vi "Get SMO Public API.vi"(8 "error in (no error)":errorcluster, 11 "Instrument.Amplifier in":refnum<class "Instrument.Amplifier.lvclass">) -> (0 "error out":errorcluster, 2 "commands":string[](array[string]), 3 "Instrument.Amplifier out":refnum<class "Instrument.Amplifier.lvclass">)   [LabVIEW 2019, in "Instrument.Amplifier.lvclass"]
doc: "Override this VI to return a list of commands supported by your Instrument"
uses:
  Instrument.Amplifier.lvclass
  Amplifier.Commands--Enum.ctl
  00ed04df-5eee-4cf2-a9f0-db2a0e5519bf.vi
  <vilib>/Utility/Data Type/Get Type Information.vi
  <vilib>/Utility/Data Type/Get Numeric Information.vi
  <userlib>/_OpenG.lib/lvdata/lvdata.llb/Unwrap VVariant__ogtk.vi
  Instrument/Instrument.lvclass
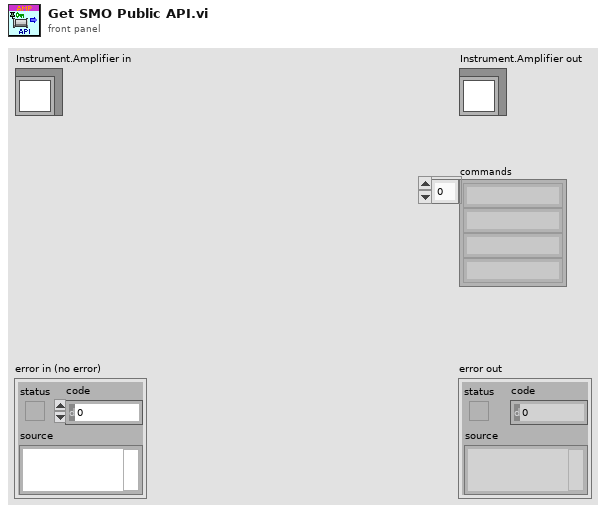
[diagram p1: front panel]
types:
  T1 = typedef "Instrument.Amplifier.lvclass/Amplifier.Commands--Enum.ctl" = enum16{"getChannel", "getAllChannels", "setChannel", "setAllChannels"}
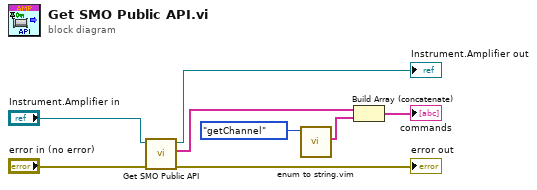
[diagram p0: block diagram]
diagram:
  n1 = call-parent "Get SMO Public API.vi"("error in (no error)"="error in (no error)", "Instrument in"="Instrument.Amplifier in") -> ("error out"=→"error out":errorcluster, "commands"=w3:string[], "Instrument out"=→"Instrument.Amplifier out":refnum<class "Instrument.Amplifier.lvclass">)  [unwired: 7 in]
  n2 = call "enum to string.vim"("enum in"=Amplifier.Commands--Enum."getChannel" ("Commands")) -> ("strings out"=w4:string[])  [unwired: 9 in, 1 out]
  n3 = Build Array (concatenate)(w3, w4) -> (→"commands":string[])
